vi "Render Picture.vi"(11 "Collection in":refnum<class "Collection.lvclass">) -> (1 "Picture":picture, 3 "Collection out":refnum<class "Collection.lvclass">)   [LabVIEW 2019, in "Collection.lvclass"]
doc: "Render the collection into the picture."
uses:
  Collection.lvclass
  Collection.lvclass/Collection.ctl
  Graphic/Graphic.lvclass
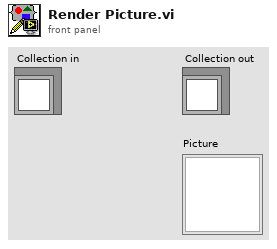
[diagram p1: front panel]
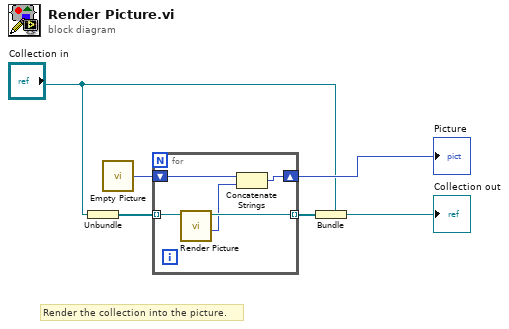
[diagram p0: block diagram]
diagram:
  # "Render the collection into the picture."
  n1 = Unbundle("Collection in") -> (w4:refnum<class "Graphic.lvclass">[])
  n2 = call "Empty Picture"() -> ("empty picture"=w2:picture)
  n3 = for {
    shift-right: [w8] -> w6
    shift-left: w2 -> [w9]
    tunnel: w4 -> [w7] mode=indexing
    tunnel: [w11] -> w3 mode=indexing
    n4 = call-dynamic "Render Picture.vi"("Graphic In"=w7) -> ("Picture"=w10:picture, "Graphic Out"=w11:refnum<class "Graphic.lvclass">)  [unwired: 9 out]
    n5 = Concatenate Strings(w9, w10) -> (w8:picture)
  }
  "Picture" <- w6
  n6 = Bundle(cluster="Collection in", w3) -> (→"Collection out":refnum<class "Collection.lvclass">)
